vi "CRYImp wiz curve construct.vi"(9 "Z strings":string[](array[string]), 10 "Y strings":string[](array[string]), 11 "X strings":string[](array[string])) -> (3 "Curve":cluster{"x":dbl, "y":dbl, "z":dbl}[](array[cluster]) {"z" format="%.2f"; "y" format="%.2f"; "x" format="%.2f"})   [LabVIEW 2013]
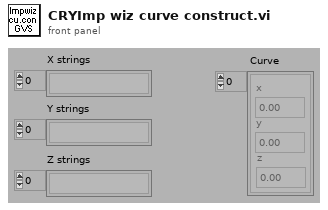
[diagram p1: front panel]
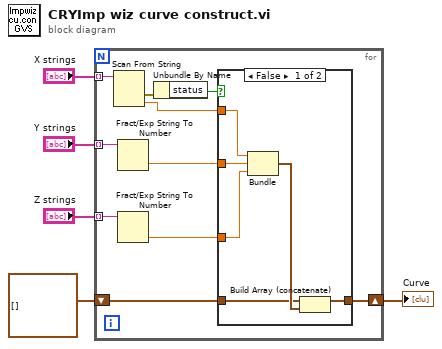
[diagram p0: block diagram]
diagram:
  n1 = for {
    shift-right: [w7] -> w1
    shift-left: cluster{"x":dbl, "y":dbl, "z":dbl}[] [] ("Curve") -> [w6]
    tunnel: "X strings" -> [w15] mode=indexing
    tunnel: "Y strings" -> [w11] mode=indexing
    tunnel: "Z strings" -> [w10] mode=indexing
    n2 = Scan From String(input string=w15) -> (error out=w14:errorcluster, output 1=w12:dbl)  [unwired: 3 in, 3 out]
    n3 = Fract/Exp String To Number(string=w11) -> (number=w9:dbl)  [unwired: 4 out]
    n4 = Fract/Exp String To Number(string=w10) -> (number=w8:dbl)  [unwired: 4 out]
    n5 = Unbundle By Name(w14) -> ("status"=w13:bool)
    n6 = case shown="False" w13 {
      tunnel: w12 -> [w20 _]
      tunnel: w9 -> [w21 _]
      tunnel: w8 -> [w19 _]
      tunnel: [w17 w22] -> w7
      tunnel: w6 -> [w16 w22]
      frame False {
        n7 = Bundle(w20, w21, w19) -> (w18:cluster{dbl, dbl, dbl})  [unwired: 1 out]
        n8 = Build Array (concatenate)(w16, w18) -> (w17:cluster{"x":dbl, "y":dbl, "z":dbl}[])
      }
      frame True {
      }
    }
  }
  "Curve" <- w1
